vi "H5LTset_attribute_string.vi"(0 "error in (no error)":errorcluster, 2 "name":string, 6 "loc_id":i32, 7 "attr_name":string, 9 "buffer":string) -> (3 "error out":errorcluster)   [LabVIEW 2009]
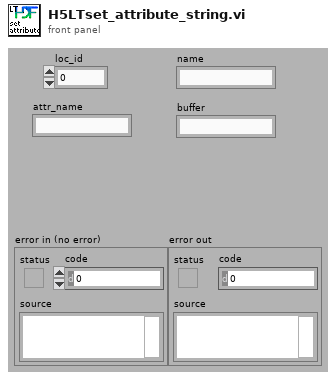
[diagram p1: front panel]
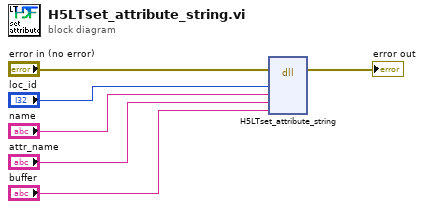
[diagram p0: block diagram]
diagram:
  n1 = dll-call lib="hdf5_hldll" fn="H5LTset_attribute_string"(error in="error in (no error)", "loc_id"="loc_id", "name"="name", "attr_name"="attr_name", "buffer"="buffer") -> (error out=→"error out":errorcluster)  [unwired: 7 in, 1 out]
